vi "decouple_modes.vi"(10 "Input":sgl[](array[numeric]) format="%#_3g") -> (2 "Decoupled":sgl[](array[numeric]) format="%#_3g")   [LabVIEW 2013]
panel:
  # "----------XY----------"
  # "----------RxRy----------"
  # "Z"
  # "Rz"
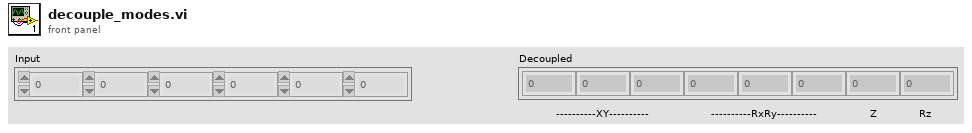
[diagram p1: front panel]
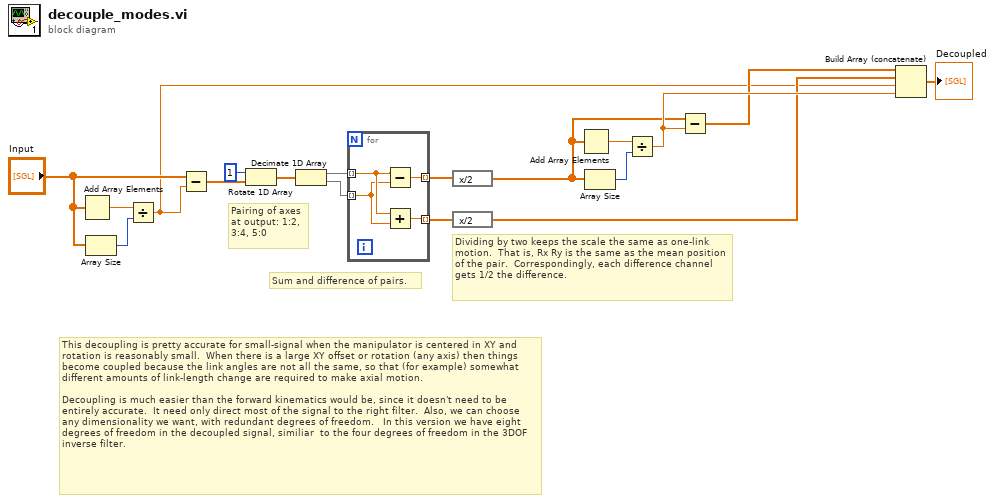
[diagram p0: block diagram]
diagram:
  # "Dividing by two keeps the scale the same as one-link motion.  That is, Rx Ry is the same as the mean position of the pair.  Correspondingly, each difference channel gets 1/2 the difference."
  # "This decoupling is pretty accurate for small-signal when the manipulator is centered in XY and rotation is reasonably small.  When there is a large XY offset or rotation (any axis) then things become coupled because the link angles are not all the same, so that (for example) somewhat different amounts of link-length change are required to make axial motion.\n\nDecoupling is much easier than the forward kinematics would be, since it doesn't need to be entirely accurate.  It need only direct most of the signal to the right filter.  Also, we can choose any dimensionality we want, with redundant degrees of freedom.   In this version we have eight  degrees of freedom in the decoupled signal, similiar  to the four degrees of freedom in the 3DOF inverse filter."
  # "Sum and difference of pairs."
  # "Pairing of axes at output: 1:2, 3:4, 5:0"
  n1 = Add Array Elements(numeric array="Input") -> (sum=w9:sgl)
  n2 = Array Size(array="Input") -> (size(s)=w10:i32)
  n3 = Divide(x=w9, y=w10) -> (x/y=w1:sgl)
  n4 = Subtract(x="Input", y=w1) -> (x-y=w12:sgl[])
  n5 = Rotate 1D Array(1:w12, 2:1 ("n")) -> (0:w14:sgl[])
  n6 = Decimate 1D Array(w14) -> (w15:sgl[], w16:sgl[])
  n7 = for {
    tunnel: w15 -> [w22] mode=indexing
    tunnel: w16 -> [w21] mode=indexing
    tunnel: [w19] -> w3 mode=indexing
    tunnel: [w20] -> w5 mode=indexing
    n8 = Subtract(x=w22, y=w21) -> (x-y=w19:sgl)
    n9 = Add(x=w22, y=w21) -> (x+y=w20:sgl)
  }
  n10 = expression code="x/2"(w3) -> (w2:sgl[])
  n11 = expression code="x/2"(w5) -> (w6:sgl[])
  n12 = Add Array Elements(numeric array=w2) -> (sum=w18:sgl)
  n13 = Array Size(array=w2) -> (size(s)=w17:i32)
  n14 = Divide(x=w18, y=w17) -> (x/y=w8:sgl)
  n15 = Subtract(x=w2, y=w8) -> (x-y=w4:sgl[])
  n16 = Build Array (concatenate)(w4, w6, w1, w8) -> (→"Decoupled":sgl[])
